vi "reset.vi"(8 "error in (no error)":errorcluster, 11 "YoutubeCacheProxy in":refnum<class "YoutubeCacheProxy.lvclass">) -> (0 "error out":errorcluster, 3 "YoutubeCacheProxy out":refnum<class "YoutubeCacheProxy.lvclass">)   [LabVIEW 2017, in "YoutubeCacheProxy.lvclass"]
uses:
  YoutubeCacheProxy.lvclass
  Globals/HashMap.ctl
  Video Class/Video.lvclass
  YoutubeCacheProxy.lvclass/YoutubeCacheProxy.ctl
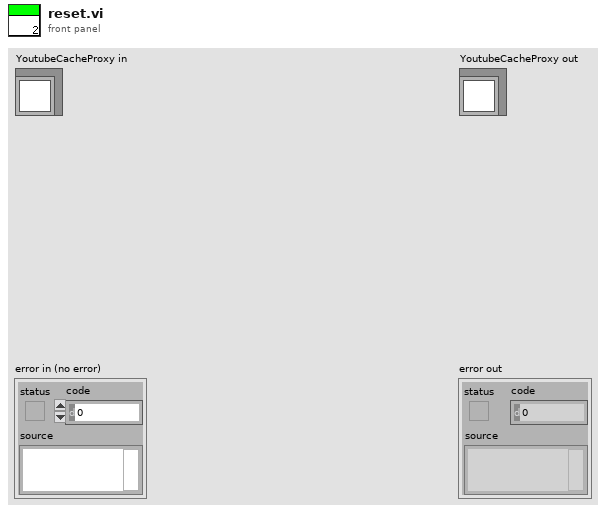
[diagram p1: front panel]
types:
  T1 = typedef "HashMap.ctl" = cluster{"Video Ids":string[], "Videos":refnum<class "Video.lvclass">[]}
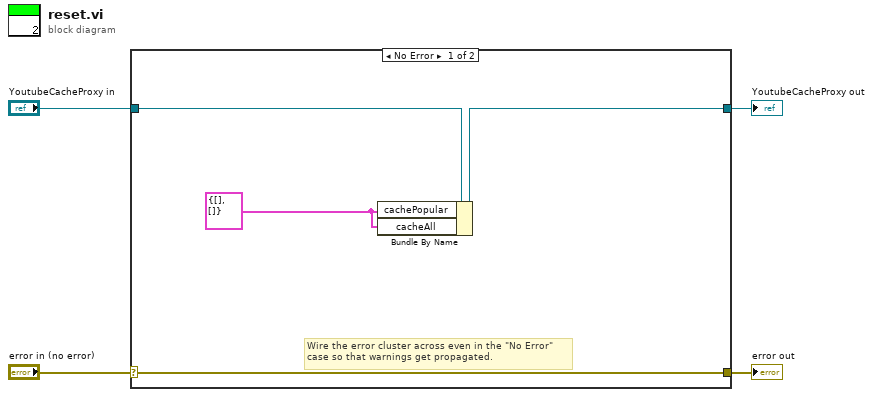
[diagram p0: block diagram]
diagram:
  n1 = case shown="No Error" "error in (no error)" {
    selector: "error in (no error)" -> [w7 w10]
    tunnel: [w7 w10] -> w3
    tunnel: [w6 w9] -> w1
    tunnel: "YoutubeCacheProxy in" -> [w8 w9]
    frame No Error {
      w5 = T1 {"Video Ids"=[], "Videos"=[]} ("HashMap")
      # "Wire the error cluster across even in the \"No Error\"\ncase so that warnings get propagated."
      n2 = Bundle By Name(cluster=w8, "cachePopular"=w5, "cacheAll"=w5) -> (w6:refnum<class "YoutubeCacheProxy.lvclass">)
    }
    frame Error {
    }
  }
  "error out" <- w3
  "YoutubeCacheProxy out" <- w1
